vi "Do.vi"(8 "error in (no error)":cluster{"状态":bool, "代码":i32, "源":string} caption="错误输入（无错误）", 10 "操作者输入":refnum<class "Actor.lvclass">, 11 "?":refnum<class "Halt Fan Msg.lvclass">) -> (0 "error out":cluster{"状态":bool, "代码":i32, "源":string} caption="错误输出", 2 "操作者输出":refnum<class "Actor.lvclass">)   [LabVIEW 2015, in "Dual Fan.lvlib" / "Halt Fan Msg.lvclass"]
uses:
  Halt Fan Msg.lvclass
  <vilib>/ActorFramework/Actor/Actor.lvclass
  Dual Fan/Dual Fan.lvclass
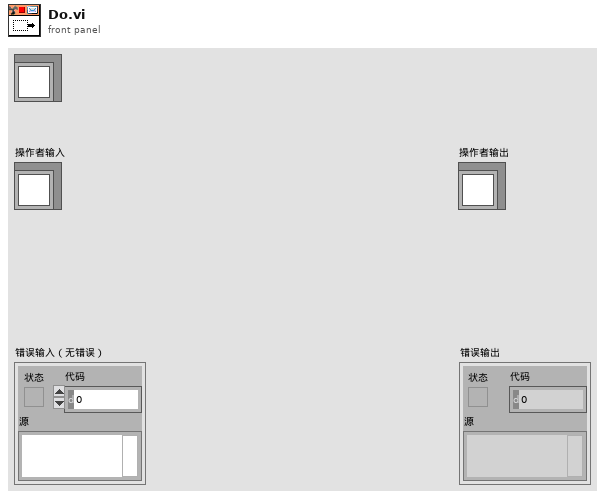
[diagram p1: front panel]
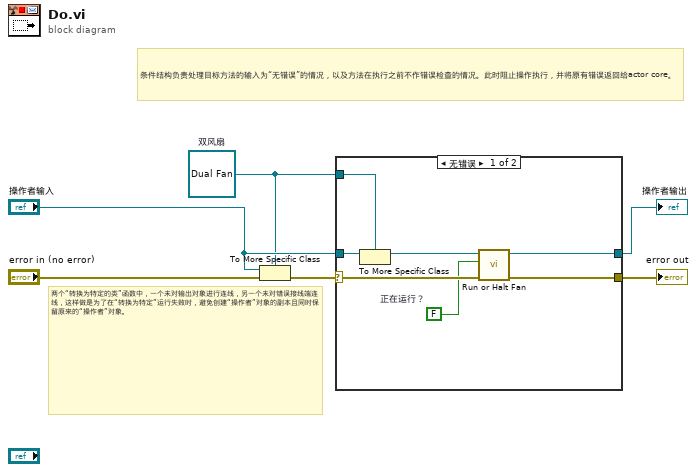
[diagram p0: block diagram]
diagram:
  w1 = refnum<class "Dual Fan.lvclass"> refnum  # 双风扇
  # "两个“转换为特定的类”函数中，一个未对输出对象进行连线，另一个未对错误接线端连线，这样做是为了在“转换为特定”运行失败时，避免创建“操作者”对象的副本且同时保留原来的“操作者”对象。"
  # "条件结构负责处理目标方法的输入为“无错误”的情况，以及方法在执行之前不作错误检查的情况。此时阻止操作执行，并将原有错误返回给actor core。"
  n1 = To More Specific Class(target class=w1, reference="操作者输入", error in="error in (no error)") -> (error out=w5:errorcluster)  [unwired: 1 out]
  n2 = case shown="无错误" w5 {
    selector: w5 -> [w8 w15]
    tunnel: [w9 w15] -> w4
    tunnel: [w10 w14] -> w3
    tunnel: "操作者输入" -> [w13 w14]
    tunnel: w1 -> [w12 _]
    frame No Error {
      w7 = FALSE  # 正在运行？
      n3 = To More Specific Class(target class=w12, reference=w13) -> (specific class reference=w11:refnum<class "Dual Fan.lvclass">)  [unwired: 1 in, 1 out]
      n4 = call "Run or Halt Fan.vi"("error in (no error)"=w8, "正在运行？"=w7, "双风扇输入"=w11) -> ("error out"=w9:cluster{"状态":bool, "代码":i32, "源":string}, "双风扇输出"=w10:refnum<class "Dual Fan.lvclass">)  [unwired: 7 in]
    }
    frame Error {
      # "如类型检查失败，则再次将原对象传出。"
    }
  }
  "error out" <- w4
  "操作者输出" <- w3
